vi "apply image perspective correction.vi"(8 "error in (no error)":errorcluster, 10 "Calibration Image":T1, 11 "Image To Correct":T1) -> (0 "error out":errorcluster, 3 "Corrected Image":T1)   [LabVIEW 2020]
uses:
  <vilib>/vision/Image Controls.llb/IMAQ Image.ctl
  <vilib>/vision/NI_Vision_Development_Module.lvlib
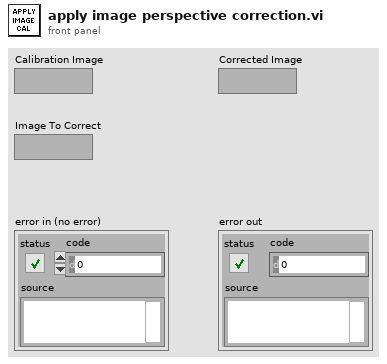
[diagram p1: front panel]
types:
  T1 = typedef "IMAQ Image.ctl" = refnum<image>
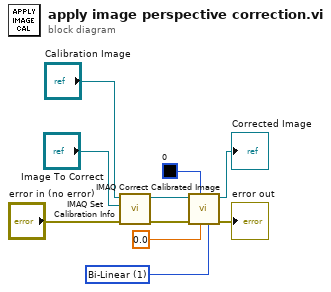
[diagram p0: block diagram]
diagram:
  w5 = u32 1 items=["Zero Order", "Bi-Linear", "Quadratic", "Cubic Spline"] ("Interpolation Type")
  n1 = call "IMAQ Set Calibration Info"("error in (no error)"="error in (no error)", "Image Dst"="Image To Correct", "Image Src"="Calibration Image") -> ("error out"=w3:errorcluster, "Calibrated Image"=w4:T1)  [unwired: 1 in, 6 out]
  n2 = call "IMAQ Correct Calibrated Image"("Interpolation Type"=w5, "Replace Value"=sgl 0.0, "Color Replace Value"=u32 0, "error in (no error)"=w3, "Image Src"=w4) -> ("error out"=→"error out":errorcluster, "Corrected Image"=→"Corrected Image":T1)  [unwired: 2 in, 3 out]
